vi "Test Timing Metrics.vi"(5 "Start?":bool, 7 "Timing Metrics In":string, 8 "Message":string) -> (1 "Timing Metrics Out":string)   [LabVIEW 2011]
uses:
  ITK/utils/strutil.llb/Case Matching.ctl
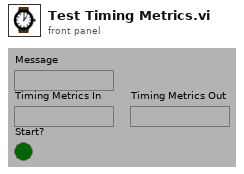
[diagram p1: front panel]
types:
  T1 = typedef "Case Matching.ctl" = enum16{"a != A", "a == A", "system"}
  T2 = typedef "Keyed Array.ctl" = cluster{"keys":string[], "values":string[]}
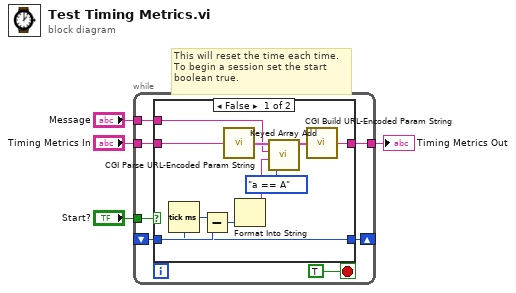
[diagram p0: block diagram]
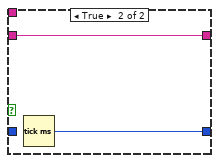
[diagram p2: hidden frame]
diagram:
  # "This will reset the time each time.\nTo begin a session set the start\nboolean true."
  n1 = while {
    tunnel: "Start?" -> [w9]
    shift-right: [w11] -> _
    shift-left: _ -> [w8]
    tunnel: "Timing Metrics In" -> [w7]
    tunnel: [w6] -> w2
    tunnel: "Message" -> [w5]
    stop <- TRUE stop-if-true
    n2 = case shown="False" w9 {
      tunnel: [w12 w23] -> w11
      tunnel: w8 -> [w14 _]
      tunnel: w7 -> [w17 w22]
      tunnel: [w16 w22] -> w6
      tunnel: w5 -> [w15 _]
      frame False {
        n3 = Tick Count (ms)() -> (millisecond timer value=w12:u32)
        n4 = Subtract(x=w12, y=w14) -> (x-y=w13:u32)
        n5 = call "CGI Parse URL-Encoded Param String.vi"("url-encoded param string"=w17) -> ("params"=w19:T2)
        n6 = Format Into String(w13) -> (resulting string=w18:string)  [unwired: 3 in, 1 out]
        n7 = call "Keyed Array Add.vi"("case matching (sensitive)"=Case_Matching."a == A", "value"=w18, "key"=w15, "array in"=w19) -> ("array out"=w21:T2)  [unwired: 3 out]
        n8 = call "CGI Build URL-Encoded Param String.vi"("params"=w21) -> ("url-encoded param string"=w16:string)
      }
      frame True {
        n9 = Tick Count (ms)() -> (millisecond timer value=w23:u32)
      }
    }
  }
  "Timing Metrics Out" <- w2
